vi "Delete_Fake_Dots_Array-3.vi"(2 "[IN] Dot matrix\nwith initial status":i16[][](array[numeric]), 3 "[IN] Source \nArray":dbl[][](array[numeric])) -> (0 "[OUT] Dot \nMatrix":i16[][](array[numeric]), 1 "[OUT] Filtered \nArray (X,Y)":dbl[][](array[numeric]))   [LabVIEW 2013]
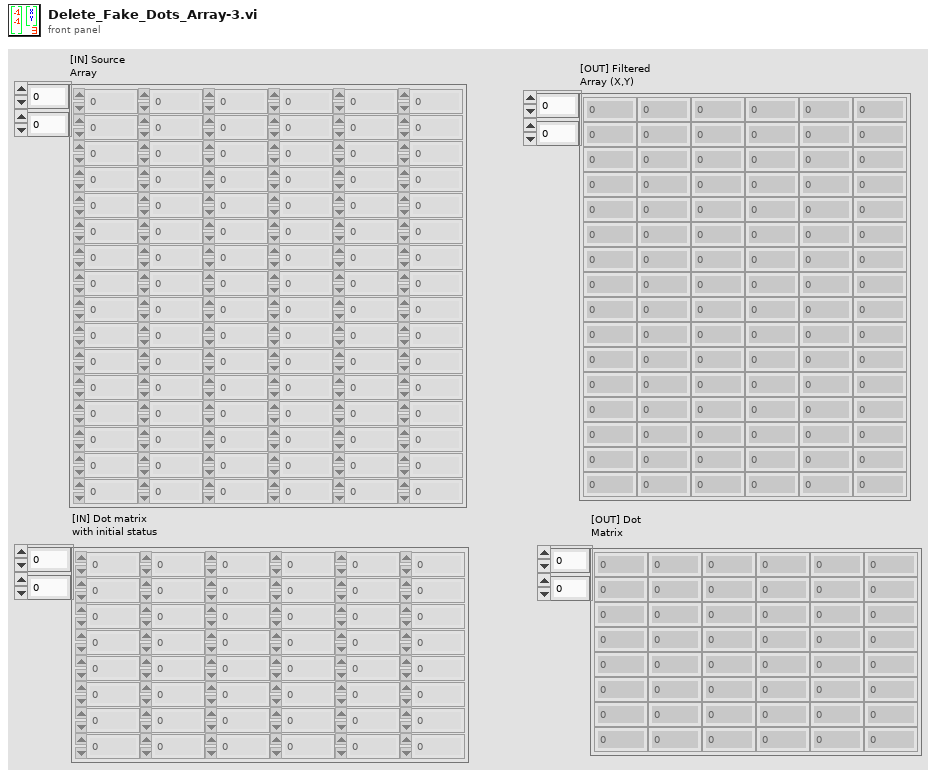
[diagram p1: front panel]
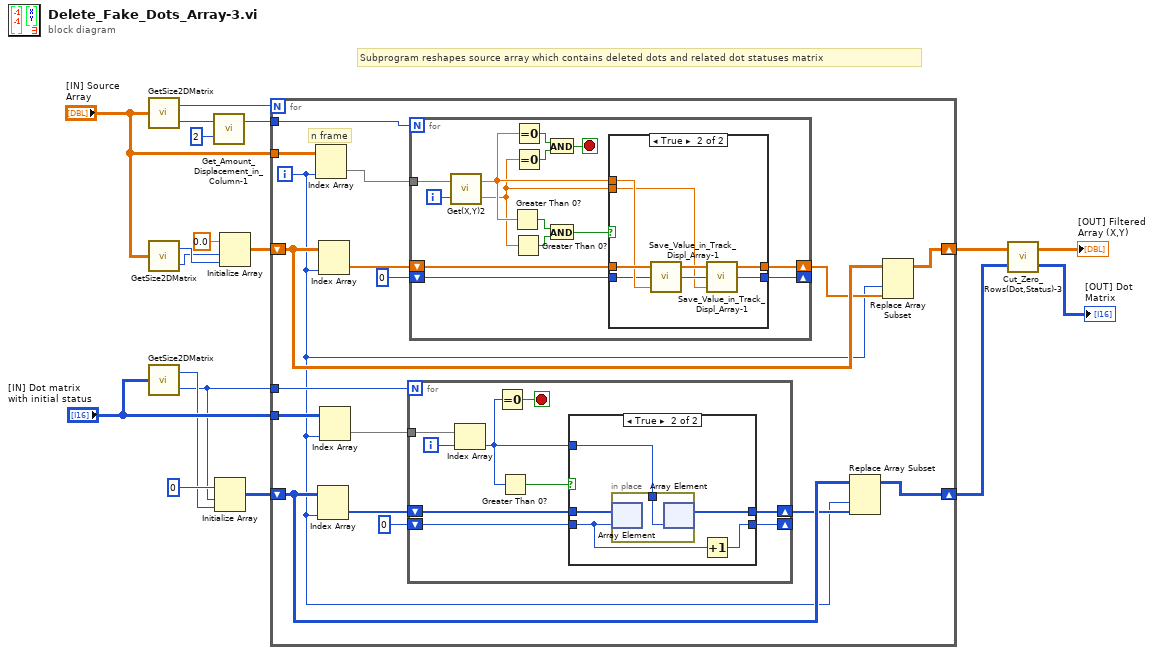
[diagram p0: block diagram]
diagram:
  # "Subprogram reshapes source array which contains deleted dots and related dot statuses matrix"
  n1 = call "GetSize2DMatrix.vi"("Array IN (2D)"="[IN] Source \nArray") -> ("# Cols"=w14:i32, "# Rows"=w12:i32)
  n2 = call "GetSize2DMatrix.vi"("Array IN (2D)"="[IN] Source \nArray") -> ("# Cols"=w17:i32, "# Rows"=w16:i32)
  n3 = call "GetSize2DMatrix.vi"("Array IN (2D)"="[IN] Dot matrix\nwith initial status") -> ("# Cols"=w7:i32, "# Rows"=w6:i32)
  n4 = call "Get_Amount_Displacement_in_Column-1.vi"("multiplier"=2 ("y"), "# Rows"=w12) -> ("Displ amount"=w10:i32)  [unwired: 1 out]
  n5 = Initialize Array(i16 0 ("element"), w6, w7) -> (w5:i16[][])
  n6 = Initialize Array(0.0 ("element"), w16, w17) -> (w15:dbl[][])
  n7 = for {
    N: w14 -> [_]
    tunnel: "[IN] Source \nArray" -> [w35]
    shift-right: [w31] -> w4
    shift-left: w15 -> [w32]
    tunnel: w10 -> [w28]
    tunnel: w6 -> [w25]
    shift-right: [w19] -> w2
    shift-left: w5 -> [w22]
    tunnel: "[IN] Dot matrix\nwith initial status" -> [w27]
    i -> [w20]
    # "n frame"
    n8 = Index Array(array=w35, index (col)=w20) -> (element=w33:dbl[])  [unwired: 1 in]
    n9 = Index Array(array=w22, index (col)=w20) -> (element=w24:i16[])  [unwired: 1 in]
    n10 = Index Array(array=w32, index (col)=w20) -> (element=w29:dbl[])  [unwired: 1 in]
    n11 = Index Array(array=w27, index (col)=w20) -> (element=w26:i16[])  [unwired: 1 in]
    n12 = for {
      N: w25 -> [_]
      tunnel: w26 -> [w44]
      shift-right: [w37] -> w21
      shift-left: w24 -> [w39]
      shift-right: [w36] -> _
      shift-left: 0 -> [w38]
      i -> [w43]
      stop <- w42 stop-if-true
      n13 = Index Array(array=w44, index=w43) -> (element=w40:i16)
      n14 = Equal To 0?(x=w40) -> (x = 0?=w42:bool)
      n15 = Greater Than 0?(x=w40) -> (x > 0?=w41:bool)
      n16 = case shown="True" w41 {
        tunnel: w40 -> [_ w48]
        tunnel: w39 -> [w46 w50]
        tunnel: w38 -> [w45 w49]
        tunnel: [w46 w47] -> w37
        tunnel: [w45 w51] -> w36
        frame False {
        }
        frame True {
          n17 = in-place {
            in-place-border: w48 -> [w52]
            n18 = in-place-array #1(w50, w49) -> ()  [unwired: 1 out]
            n19 = in-place-array #1(w52) -> (w47:i16[])  [unwired: 1 out]
          }
          n20 = Increment(x=w49) -> (x+1=w51:i32)
        }
      }
    }
    n21 = for {
      N: w28 -> [_]
      tunnel: w33 -> [w56]
      shift-right: [w57] -> w30
      shift-left: w29 -> [w60]
      shift-right: [w58] -> _
      shift-left: 0 -> [w59]
      i -> [w55]
      stop <- w64 stop-if-true
      n22 = call "Get(X,Y)2.vi"("[IN] index of (X,Y)"=w55, "[IN] Array coordi\nnates (X,Y) in Frame"=w56) -> ("[OUT] Y"=w53:dbl, "[OUT] X"=w54:dbl)
      n23 = Greater Than 0?(x=w54) -> (x > 0?=w63:bool)
      n24 = Greater Than 0?(x=w53) -> (x > 0?=w62:bool)
      n25 = Equal To 0?(x=w54) -> (x = 0?=w66:bool)
      n26 = Equal To 0?(x=w53) -> (x = 0?=w65:bool)
      n27 = And(x=w66, y=w65) -> (x .and. y?=w64:bool)
      n28 = And(x=w63, y=w62) -> (x .and. y?=w61:bool)
      n29 = case shown="True" w61 {
        tunnel: w60 -> [w68 w76]
        tunnel: w59 -> [w67 w74]
        tunnel: w54 -> [_ w75]
        tunnel: w53 -> [_ w69]
        tunnel: [w67 w70] -> w58
        tunnel: [w68 w72] -> w57
        frame False {
        }
        frame True {
          n30 = call "Save_Value_in_Track_Displ_Array-1.vi"("[IN] Value"=w75, "[IN] Index"=w74, "[IN] Empty tracks\nfor points saving"=w76) -> ("[OUT] Index ++"=w71:i32, "[OUT Track with saved value"=w73:dbl[])  [unwired: 1 in]
          n31 = call "Save_Value_in_Track_Displ_Array-1.vi"("[IN] Value"=w69, "[IN] Index"=w71, "[IN] Empty tracks\nfor points saving"=w73) -> ("[OUT] Index ++"=w70:i32, "[OUT Track with saved value"=w72:dbl[])  [unwired: 1 in]
        }
      }
    }
    n32 = Replace Array Subset(array=w22, new element=w21, index (col)=w20) -> (w19:i16[][])  [unwired: 1 in]
    n33 = Replace Array Subset(array=w32, new element=w30, index (col)=w20) -> (w31:dbl[][])  [unwired: 1 in]
  }
  n34 = call "Cut_Zero_Rows(Dot,Status)-3.vi"("[IN] Dot matrix\nwith zero points"=w2, "Array (X,Y) IN"=w4) -> ("[OUT] Dot \nMatrix"=→"[OUT] Dot \nMatrix":i16[][], "Array (X,Y) OUT"=→"[OUT] Filtered \nArray (X,Y)":dbl[][])
